vi "U32.vi"(1 "Numeric Input":u32) -> (0 "Numeric Output":u32)   [LabVIEW 2013]
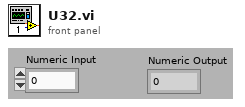
[diagram p1: front panel]
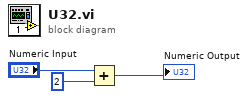
[diagram p0: block diagram]
diagram:
  n1 = Add(x="Numeric Input", y=u32 2) -> (x+y=→"Numeric Output":u32)
